vi "Motor FGV.vi"(9 "Direction":enum16{"CW", "CCW"}(ring), 10 "Type":enum16{"Full", "Half", "Torque"}(ring), 11 "Action":enum16{"Reset", "Set", "Get"}(ring)) -> (3 "Coil state":bool[](array[boolean]))   [LabVIEW 2020]
panel:
  # "Action: \n- Reset: outputs an array of zeroes\n- Set: defines sequences by type and direction\n-Get: cycles though the defined sequence"
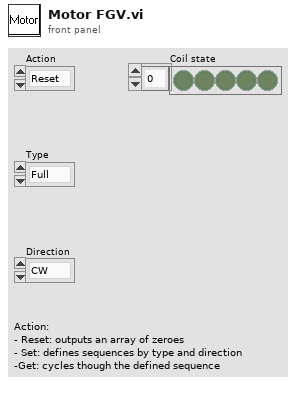
[diagram p1: front panel]
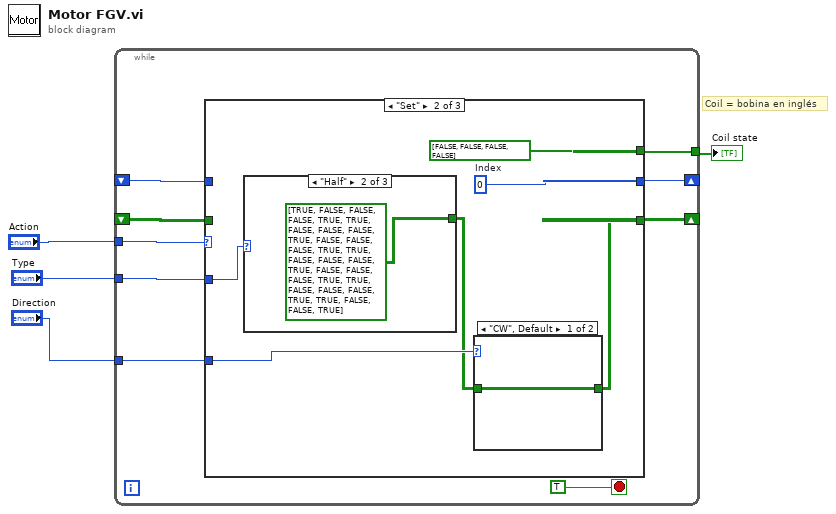
[diagram p0: block diagram]
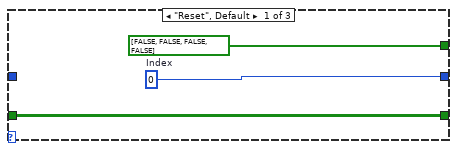
[diagram p2: hidden frame]
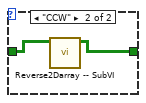
[diagram p3: hidden frame]
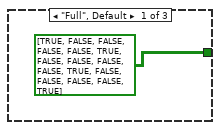
[diagram p4: hidden frame]
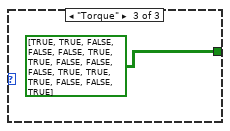
[diagram p5: hidden frame]
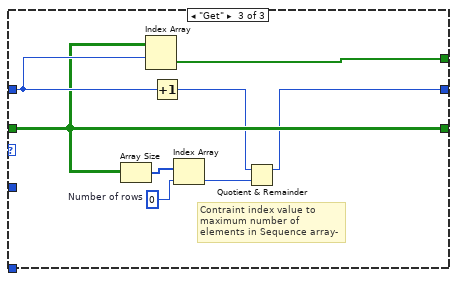
[diagram p6: hidden frame]
diagram:
  # "Coil = bobina en inglés"
  n1 = while {
    tunnel: "Action" -> [w12]
    tunnel: [w10] -> w3
    tunnel: "Type" -> [w11]
    shift-right: [w9] -> _
    shift-left: _ -> [w8]
    shift-right: [w7] -> _
    shift-left: _ -> [w6]
    tunnel: "Direction" -> [w5]
    stop <- TRUE ("stop") stop-if-true
    n2 = case shown="\"Set\"" w12 {
      tunnel: [w15 w17 w34] -> w9
      tunnel: w11 -> [_ w22 _]
      tunnel: [bool[] [FALSE, FALSE, FALSE, FALSE] bool[] [FALSE, FALSE, FALSE, FALSE] w36] -> w10
      tunnel: w8 -> [w15 _ w34]
      tunnel: [w14 w20 w29] -> w7
      tunnel: w6 -> [_ _ w35]
      tunnel: w5 -> [_ w19 _]
      frame "Reset", Default {
        w14 = 0  # Index
      }
      frame "Set" {
        w20 = 0  # Index
        n3 = case shown="\"Half\"" w22 {
          tunnel: [bool[][] [[TRUE, FALSE, FALSE, FALSE], [FALSE, TRUE, FALSE, FALSE], [FALSE, FALSE, TRUE, FALSE], [FALSE, FALSE, FALSE, TRUE]] bool[][] [[TRUE, FALSE, FALSE, FALSE], [TRUE, TRUE, FALSE, FALSE], [FALSE, TRUE, FALSE, FALSE], [FALSE, TRUE, TRUE, FALSE], [FALSE, FALSE, TRUE, FALSE], [FALSE, FALSE, TRUE, TRUE], [FALSE, FALSE, FALSE, TRUE], [TRUE, FALSE, FALSE, TRUE]] bool[][] [[TRUE, TRUE, FALSE, FALSE], [FALSE, TRUE, TRUE, FALSE], [FALSE, FALSE, TRUE, TRUE], [TRUE, FALSE, FALSE, TRUE]]] -> w18
          frame "Full", Default {
          }
          frame "Half" {
          }
          frame "Torque" {
          }
        }
        n4 = case shown="\"CW\", Default" w19 {
          tunnel: w18 -> [w23 w25]
          tunnel: [w23 w24] -> w17
          frame "CW", Default {
          }
          frame "CCW" {
            n5 = call "Reverse2Darray -- SubVI.vi"("Input Array"=w25) -> ("Reverse Array"=w24:bool[][])  [unwired: 10 in]
          }
        }
      }
      frame "Get" {
        w32 = 0  # Number of rows
        # "Contraint index value to \nmaximum number of \nelements in Sequence array-"
        n6 = Array Size(array=w34) -> (size(s)=w33:i32[])
        n7 = Index Array(array=w34, index (row)=w35) -> (element=w36:bool[])  [unwired: 1 in]
        n8 = Increment(x=w35) -> (x+1=w31:i32)
        n9 = Index Array(array=w33, index=w32) -> (element=w30:i32)
        n10 = Quotient & Remainder(x=w31, y=w30) -> (x-y*floor(x/y)=w29:i32)  [unwired: 1 out]
      }
    }
  }
  "Coil state" <- w3
